vi "Destroy.vi"(8 "error in (no error)":errorcluster, 11 "reference in":refnum<class "Camera_Sim.lvclass">) -> (0 "error out":errorcluster, 3 "reference out":refnum<class "Camera_Sim.lvclass">)   [LabVIEW 2017, in "Camera_Sim.lvclass"]
uses:
  Camera_Sim.lvclass
  Camera_class/Camera.lvclass
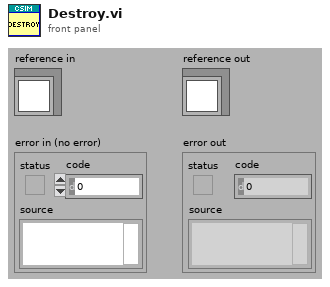
[diagram p1: front panel]
types:
  T1 = typedef "Camera_Sim.lvclass/ObjectAttributes.ctl" = cluster{"Connected":bool, "Image Out":T2, "Frame Number":u32, "Image Directory":path, "Images in Directory":path[]}
  T2 = typedef "IMAQ Image.ctl" = refnum<image>
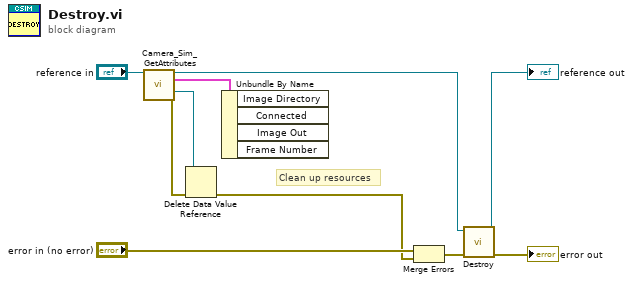
[diagram p0: block diagram]
diagram:
  # "Clean up resources"
  n1 = call "Camera_Sim_GetAttributes.vi"("reference in"="reference in") -> ("reference out"=w3:refnum<class "Camera_Sim.lvclass">, "Data"=w9:T1, "DataRef"=w8:refnum<data-value>, "error out"=w10:errorcluster)  [unwired: 11 in]
  n2 = Delete Data Value Reference(data value reference=w8, error in=w10) -> (error out=w6:errorcluster)  [unwired: 1 out]
  n3 = Unbundle By Name(w9) -> ()  [unwired: 4 out]
  n4 = Merge Errors("error in (no error)", w6) -> (w4:errorcluster)
  n5 = call-parent "Destroy.vi"("error in (no error)"=w4, "reference in"=w3) -> ("error out"=→"error out":errorcluster, "reference out"=→"reference out":refnum<class "Camera_Sim.lvclass">)  [unwired: 8 in]
